vi "Задание_АБ_расп._Рэлея.vi"() -> ()   [LabVIEW 2017]
uses:
  <vilib>/Analysis/baseanly.llb/Mean (DBL).vi
  <vilib>/gmath/statdist.llb/Beta Random.vi
  <vilib>/Analysis/3filter.llb/Bessel Filter (DBL).vi
  <vilib>/Analysis/NI_AALBase.lvlib
  <vilib>/gmath/NI_Gmath.lvlib
panel:
  out "Шум на основе распределения Рэлея":dbl[](graph)
  out "Итого. кол-во бит":i32
  in  "Пороговое значение":dbl
  out "Демодулированный и отфильтрованный сигнал":dbl[][](graph)
  out "Демодулированный сигнал":i16[](graph)
  in  "Нижняя частота среза":dbl
  in  "Порядок фильтра":i64(slide) scale=0.0..20.0
  in  "Переменная floor(x/y)":i32
  out "Модулирующий сигнал":dbl[](graph)
  out "Частотно модулированный цифровой сигнал":dbl[](graph)
  in  "см. 1.2 Циклов в секунду":i32(slide) scale=4.0..50.0
  in  "Сколько битов брать":i32=4
  out "Радио сигнал с паузами":dbl[](graph)
  in  "Кол-во выборок":i32=400
  out "Массив с паузами":dbl[](array[numeric])
  in  "Количество бит":i32=8
  out "Вырезка из массива":dbl[](array[numeric])
  out "Биты на выходе 1":dbl[](array[numeric])
  # "Демодуляция"
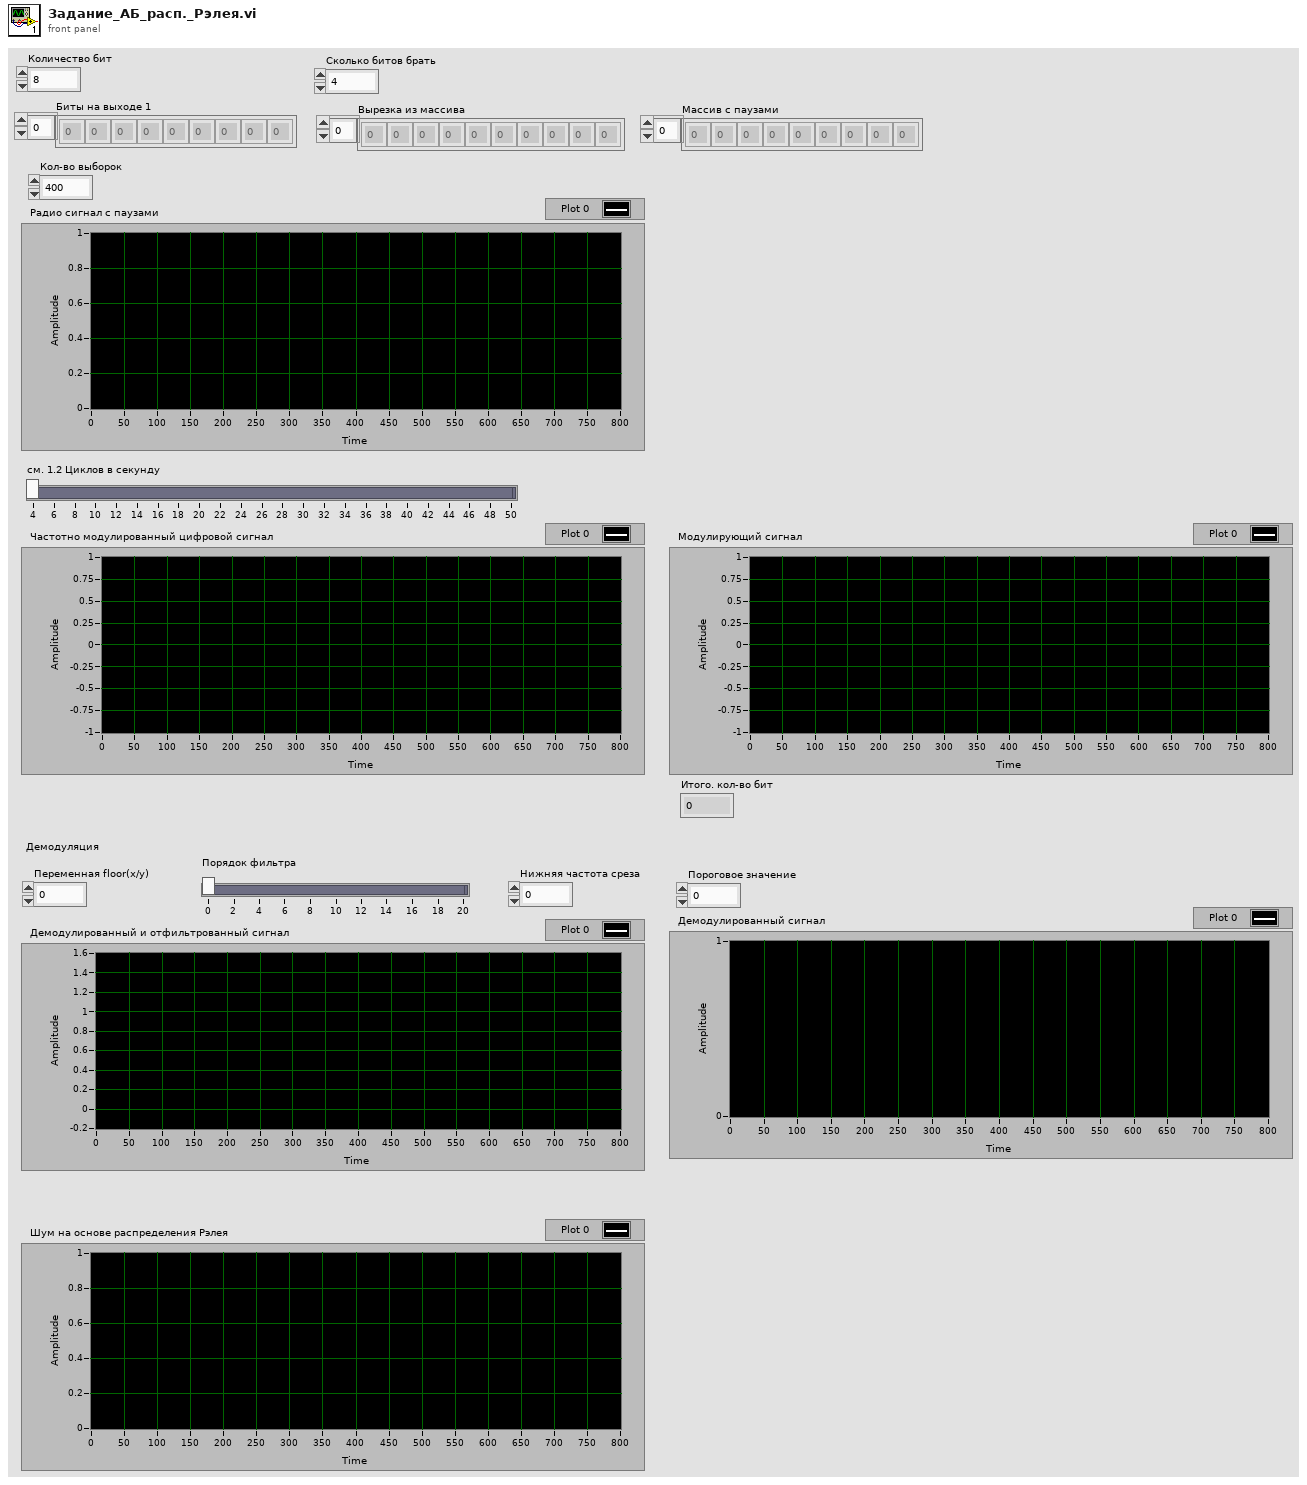
[diagram p1: front panel]
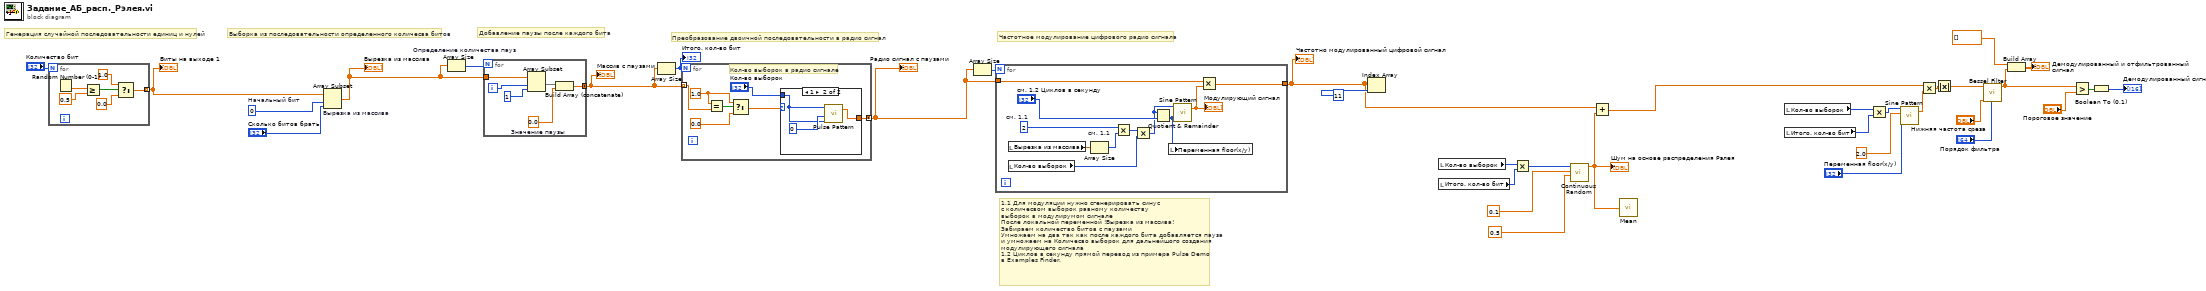
[diagram p0: block diagram]
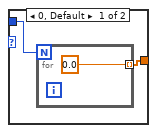
[diagram p2: hidden frame]
diagram:
  w34 = 0  # Начальный бит
  # "1.1 Для модуляции нужно сгенерировать синус \nс количесвом выборок равному количеству \nвыборок в модулирумом сигнале\nПосле локальной переменной !Вырезка из массива! \nЗабираем количество битов с паузами \nУмножаем на два так как после каждого бита добавляется пауза\nи умножаем на Количесво выборок для дальнейшого создания  \nмодулирующего сигнала\n1.2 Циклов в секунду прямой перевод из примера Pulse Demo \nв Examples Finder."
  # "Преобразование двоичной последовательности в радио сигнал"
  # "Частотное модулирование цифрового радио сигнала"
  # "Добавление паузы после каждого бита"
  # "Выборка из последовательности определенного количесва битов"
  # "Генерация случайной последовательности единиц и нулей"
  n1 = for {
    N: "Количество бит" -> [_]
    tunnel: [w36] -> w32 mode=indexing
    n2 = Random Number (0-1)() -> (number: 0 to 1=w41:dbl)
    n3 = Greater Or Equal?(x=w41, y=0.5) -> (x >= y?=w39:bool)
    n4 = Select(t=1.0, s=w39, f=0.0) -> (s? t:f=w36:dbl)
  }
  "Биты на выходе 1" <- w32
  n5 = Array Subset "Вырезка из массива"(array=w32, index=w34, length="Сколько битов брать") -> (w30:dbl[])
  "Вырезка из массива" <- w30
  n6 = Array Size "Определение количества пауз"(array=w30) -> (size(s)=w31:i32)
  n7 = for {
    N: w31 -> [_]
    tunnel: w30 -> [w44]
    tunnel: [w43] -> w27 mode=concatenating
    i -> [w42]
    w45 = 0.0  # Значение паузы
    n8 = Array Subset(array=w44, index=w42, length=1) -> (w46:dbl[])
    n9 = Build Array (concatenate)(w46, w45) -> (w43:dbl[])
  }
  "Массив с паузами" <- w27
  n10 = Array Size(array=w27) -> (size(s)=w28:i32)
  "Итого. кол-во бит" <- w28
  n11 = for {
    N: w28 -> [_]
    tunnel: w27 -> [w51] mode=indexing
    tunnel: [w49] -> w26 mode=concatenating
    w53 = 1.0
    # "Кол-во выборок в радио сигнале"
    n12 = Equal?(x=w53, y=w51) -> (x = y?=w54:bool)
    n13 = Select(t=w53, s=w54, f=0.0) -> (s? t:f=w50:dbl)
    n14 = case shown="1" w50 {
      tunnel: [w55 w59] -> w49
      tunnel: "Кол-во выборок" -> [w56 w58]
      frame 0, Default {
        n15 = for {
          N: w56 -> [_]
          tunnel: [0.0] -> w55 mode=indexing
        }
      }
      frame 1 {
        n16 = call <vilib>:"Pulse Pattern.vi"("width"=w58, "delay"=0, "samples"=w58) -> ("Pulse Pattern"=w59:dbl[])  [unwired: 1 in, 1 out]
      }
    }
  }
  "Радио сигнал с паузами" <- w26
  n17 = Array Size(array=w26) -> (size(s)=w29:i32)
  n18 = for {
    N: w29 -> [_]
    tunnel: w26 -> [w70]
    tunnel: [w69] -> w2
    w65 = 2  # см. 1.1
    n19 = local read "Вырезка из массива"() -> (w67:dbl[])
    n20 = local read "Кол-во выборок"() -> (w63:i32)
    n21 = Array Size "см. 1.1"(array=w67) -> (size(s)=w66:i32)
    n22 = Multiply(x=w65, y=w66) -> (x*y=w64:i32)
    n23 = Multiply(x=w64, y=w63) -> (x*y=w62:i32)
    n24 = Quotient & Remainder(x=w62, y="см. 1.2 Циклов в секунду") -> (floor(x/y)=w61:i32)  [unwired: 1 out]
    n25 = local write "Переменная floor(x/y)"(w61) -> ()
    n26 = call <vilib>:"Sine Pattern.vi"("cycles"=w61, "samples"=w62) -> ("Sinusoidal Pattern"=w68:dbl[])  [unwired: 2 in, 1 out]
    "Модулирующий сигнал" <- w68
    n27 = Multiply(x=w70, y=w68) -> (x*y=w69:dbl[])
  }
  "Частотно модулированный цифровой сигнал" <- w2
  n28 = Index Array(array=w2, index=11 ("index (row)")) -> ()  [unwired: 1 out]
  n29 = local read "Кол-во выборок"() -> (w6:i32)
  n30 = local read "Итого. кол-во бит"() -> (w5:i32)
  n31 = Multiply(x=w6, y=w5) -> (x*y=w4:i32)
  n32 = call-poly <vilib>:"Continuous Random.vi"("b"=0.5, "a"=0.1 ("x"), "samples"=w4) -> ("beta random data"=w3:dbl[])  [unwired: 7 in, 1 out]
  "Шум на основе распределения Рэлея" <- w3
  n33 = Add(x=w2, y=w3) -> (x+y=w1:dbl[])
  n34 = call-poly <vilib>:"Mean.vi"("X"=w3) -> ()  [unwired: 2 out]
  n35 = local read "Кол-во выборок"() -> (w10:i32)
  n36 = local read "Итого. кол-во бит"() -> (w9:i32)
  n37 = Multiply(x=w10, y=w9) -> (x*y=w11:i32)
  n38 = call <vilib>:"Sine Pattern.vi"("cycles"="Переменная floor(x/y)", "amplitude"=2.0, "samples"=w11) -> ("Sinusoidal Pattern"=w13:dbl[])  [unwired: 1 in, 1 out]
  n39 = Multiply(x=w1, y=w13) -> (x*y=w22:dbl[])
  n40 = Absolute Value(x=w22) -> (abs(x)=w19:dbl[])
  n41 = call-poly <vilib>:"Bessel Filter.vi"("order"="Порядок фильтра", "low cutoff freq: fl"="Нижняя частота среза", "X"=w19) -> ("Filtered X"=w17:dbl[])  [unwired: 5 in, 1 out]
  n42 = Build Array(dbl[] [] ("element"), w17) -> (→"Демодулированный и отфильтрованный сигнал":dbl[][])
  n43 = Greater?(x=w17, y="Пороговое значение") -> (0:w16:bool[])
  n44 = Boolean To (0,1)(Boolean=w16) -> (0, 1=→"Демодулированный сигнал":i16[])
